vi "FGV-GEvt Filter Rules(lvlibp).vi"(6 "Set? (T)/Get(F)":bool, 8 "Error In":errorcluster caption="error in (no error)", 11 "Rules-v1":T1) -> (0 "error out":errorcluster, 3 "Rules-v1":T1)   [LabVIEW 2017, in "Communicable State Machine.lvlib"]
uses:
  Communicable State Machine.lvlib
  Typedef/_CSM_GlobalLog Filter Rules - v1.0.ctl
  Typedef/_CSM_GlobalLog_MSG_TYPE.ctl
  Typedef/_CSM_GlobalLog_STATE_TYPE.ctl
  _Shared/CSM Shared.lvlib
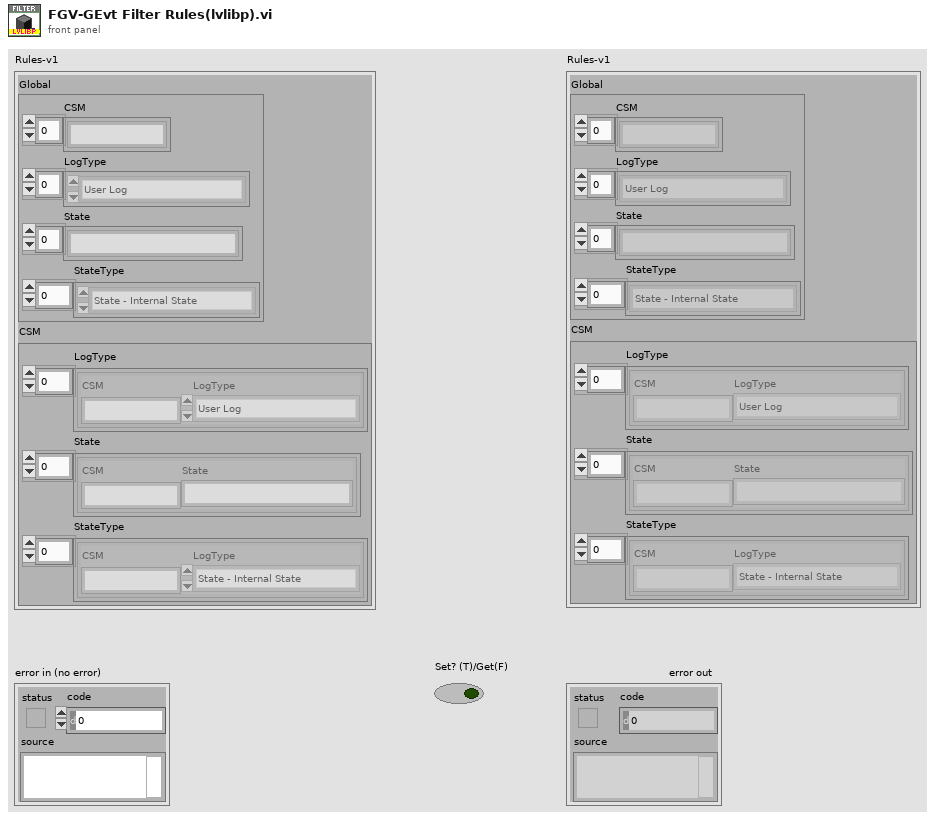
[diagram p1: front panel]
types:
  T1 = typedef "Communicable State Machine.lvlib/_CSM_GlobalLog Filter Rules - v1.0.ctl" = cluster{"Global":cluster{"CSM":string[], "LogType":T2[], "State":string[], "StateType":T3[]}, "CSM":cluster{"LogType":cluster{"CSM":string, "LogType":T2}[], "State":cluster{"CSM":string, "State":string}[], "StateType":cluster{"CSM":string, "LogType":T3}[]}}
  T2 = typedef "Communicable State Machine.lvlib/_CSM_GlobalLog_MSG_TYPE.ctl" = enum16{"User Log", "State Change", "Status", "Interrupt", "Register", "Unregister", "Error Log", "Module Created", "Module Destroyed", "Async Message", "No-Rep Async Message", "Sync Message"}
  T3 = typedef "Communicable State Machine.lvlib/_CSM_GlobalLog_STATE_TYPE.ctl" = enum16{"State - Internal State", "State - External Message", "State - Response", "State - Complete"}
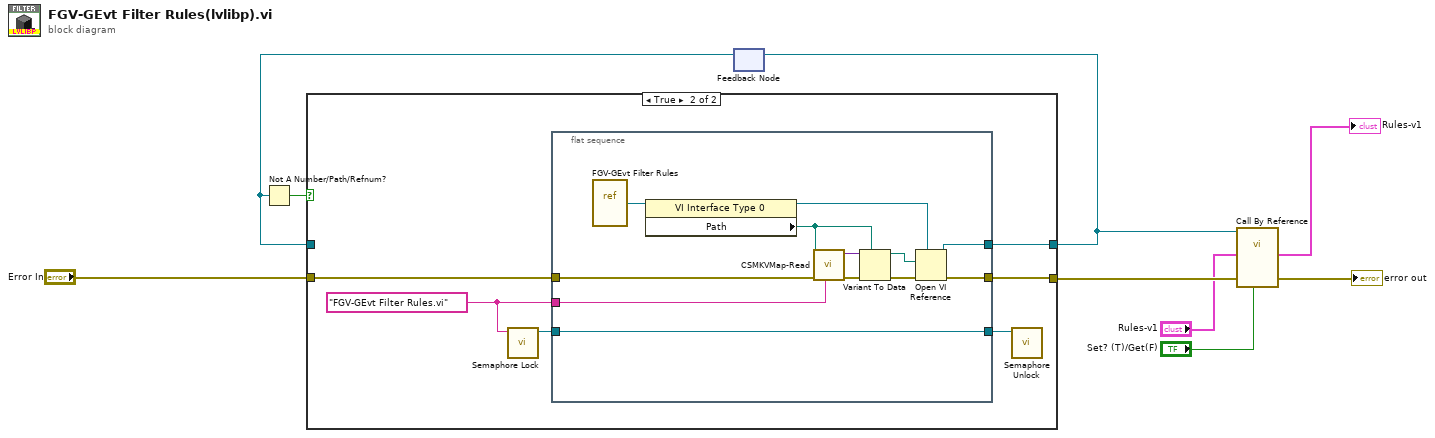
[diagram p0: block diagram]
diagram:
  n1 = feedback #1() -> (w8:refnum<vi>)  [unwired: 1 in]
  n2 = Not A Number/Path/Refnum?(number/path/refnum=w8) -> (NaN/Path/Refnum?=w9:bool)
  n3 = case shown="True" w9 {
    tunnel: [w10 w16] -> w7
    tunnel: [w11 w17] -> w6
    tunnel: "Error In" -> [w11 w15]
    tunnel: w8 -> [w10 _]
    frame False {
    }
    frame True {
      w14 = "FGV-GEvt Filter Rules.vi" ("name")
      n4 = call "Semaphore Lock.vi"("name"=w14) -> ("semaphore"=w13:refnum<queue>)  [unwired: 10 in]
      n5 = flat-sequence {
        tunnel: [w25] -> w17
        tunnel: [w23] -> w16
        tunnel: w15 -> [w21]
        tunnel: w14 -> [w19]
        tunnel: w13 -> [w18]
        tunnel: [w18] -> w12
        frame #0 {
          n6 = vi-ref "FGV-GEvt Filter Rules.vi"() -> (w20:refnum<vi>)
          n7 = property class="VI Interface Type 0"(reference=w20) -> (reference out=w22:refnum<vi>, "Path"=w24:path)  [unwired: 1 in, 1 out]
          n8 = call "CSMKVMap-Read.vi"("name"=w19, "Error in"=w21, "default value (empty variant)"=w24) -> ("Error out"=w29:errorcluster, "value"=w28:variant)  [unwired: 5 in]
          n9 = Variant To Data(error in=w29, type=w24, Variant=w28) -> (data=w27:path, error out=w26:errorcluster)
          n10 = Open VI Reference(type specifier VI Refnum (for type only)=w22, vi path=w27, error in (no error)=w26) -> (vi reference=w23:refnum<vi>, error out=w25:errorcluster)  [unwired: 3 in]
        }
      }
      n11 = call "Semaphore Unlock.vi"("semaphore"=w12) -> ()  [unwired: 11 in]
    }
  }
  n12 = feedback-in #1(w7) -> ()
  n13 = call-by-ref "?"(reference=w7, "Set? (T)/Get(F)"="Set? (T)/Get(F)", "Error In"=w6, "Rules-v1"="Rules-v1") -> ("error out"=→"error out":errorcluster, "Rules-v1"=→"Rules-v1":T1)  [unwired: 8 in, 2 out]
